vi "exnSpectralBlock spectral measurements PSD WFM.vi"(0 "Signals":waveform(dbl)(graph), 5 "Restart Averaging":bool, 7 "View":T2, 9 "Spectrum Window":u16, 11 "error in (no error)":errorcluster, 12 "Spectrum Averaging Parameters":T1={"averaging mode"=0, "weighting mode"=1, "number of averages"=10} {"averaging mode" items=["No averaging", "Vector averaging", "RMS averaging", "Peak hold"]; "weighting mode" items=["Linear", "Exponential"]}, 14 "All Spectra":bool) -> (4 "Measurement Output":cluster{"f0":dbl, "df":dbl, "magnitude":dbl[]}(graph), 6 "averaging done":bool, 15 "error out":errorcluster)   [LabVIEW 2020]
uses:
  <vilib>/measure/NI_MAPro.lvlib
panel:
  in  "time signal":waveform(dbl)
  in  "measurement":string="PSD"
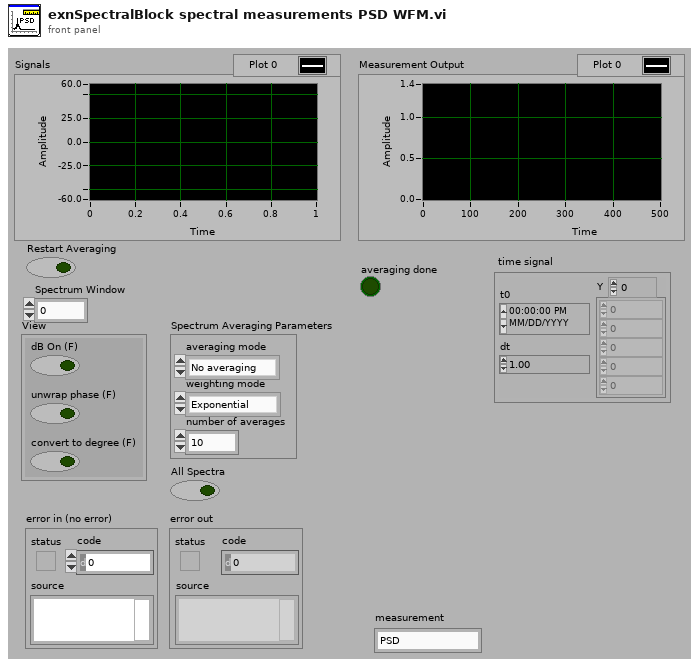
[diagram p1: front panel]
types:
  T1 = cluster{"averaging mode":u16, "weighting mode":u16, "number of averages":u32}
  T2 = cluster{"dB On (F)":bool, "unwrap phase (F)":bool, "convert to degree (F)":bool}
  T3 = enum16{"None ", "Hanning", "Hamming", "Blackman-Harris", "Exact Blackman", "Blackman", "Flat Top", "4 Term B-Harris ", "7 Term B-Harris", "Low Sidelobe"}
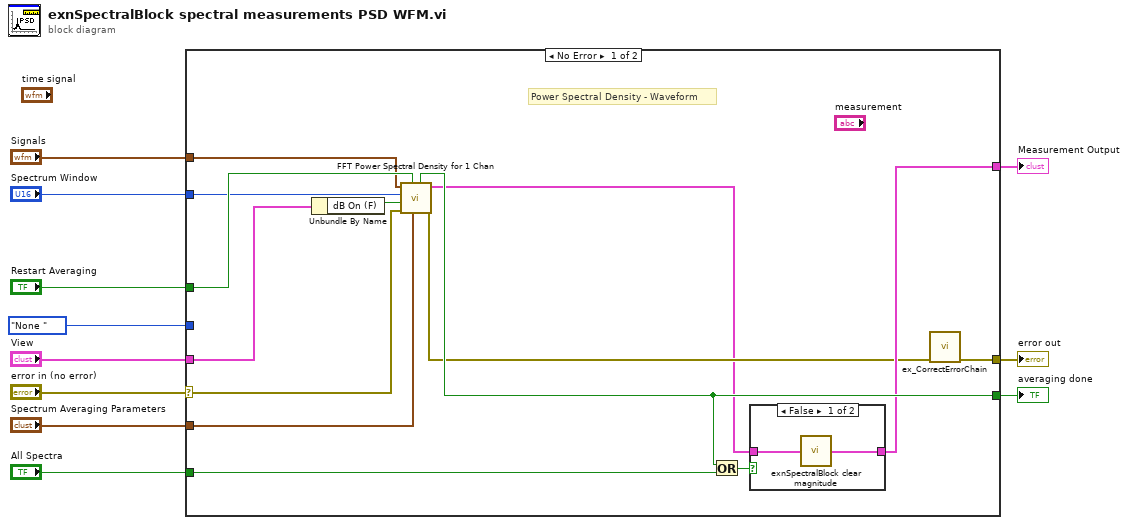
[diagram p0: block diagram]
diagram:
  n1 = case shown="No Error" "error in (no error)" {
    selector: "error in (no error)" -> [w17 w29]
    tunnel: [w14 _] -> w11
    tunnel: [w25 _] -> w10
    tunnel: "All Spectra" -> [w24 _]
    tunnel: "Spectrum Averaging Parameters" -> [w23 _]
    tunnel: "Restart Averaging" -> [w22 _]
    tunnel: T3."None " ("window") -> [_ _]
    tunnel: "Spectrum Window" -> [w18 _]
    tunnel: "View" -> [w21 _]
    tunnel: "Signals" -> [w15 _]
    tunnel: [w20 w29] -> w4
    frame No Error {
      # "Power Spectral Density - Waveform"
      n2 = Unbundle By Name(w21) -> ("dB On (F)"=w16:bool)
      n3 = call <vilib>:"FFT Power Spectral Density for 1 Chan.vi"("averaging parameters"=w23, "restart averaging (F)"=w22, "error in (no error)"=w17, "dB On (F)"=w16, "window"=w18, "time signal"=w15) -> ("error out"=w13:errorcluster, "power spectral density"=w12:cluster{"f0":dbl, "df":dbl, "magnitude":dbl[]}, "averaging done"=w25:bool)  [unwired: 2 in, 1 out]
      n4 = Or(x=w25, y=w24) -> (x .or. y?=w19:bool)
      n5 = case shown="False" w19 {
        tunnel: w12 -> [w27 w28]
        tunnel: [w26 w28] -> w14
        frame False {
          n6 = call <vilib>:"exnSpectralBlock clear magnitude.vi"("magnitude in"=w27) -> ("magnitude out"=w26:cluster{"f0":dbl, "df":dbl, "magnitude":dbl[]})
        }
        frame True {
        }
      }
      n7 = call <vilib>:"ex_CorrectErrorChain.vi"("error in (no error)"=w13) -> ("error out"=w20:errorcluster)  [unwired: 10 in]
    }
    frame Error {
    }
  }
  "Measurement Output" <- w11
  "averaging done" <- w10
  "error out" <- w4
